vi "Run 03.vi"(11 "NXT/EV3 in":T1) -> (3 "EV3 out":T1)   [LabVIEW 2016]
uses:
  <vilib>/NXT/Subs/LVHSConnector.ctl
  <vilib>/NXT/LegoClasses/BrickReference/BrickReference.lvclass
  <vilib>/NXT/Block Support/NXT_ButtonSelector.ctl
  <vilib>/NXT/Dual Mode Library/Waits/Wait_Btn_Press.vi
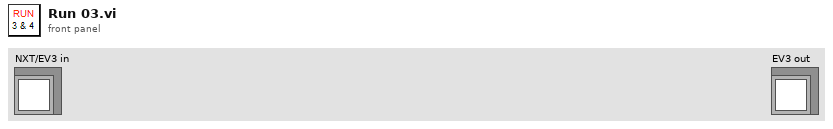
[diagram p1: front panel]
types:
  T1 = typedef "LVHSConnector.ctl" = refnum<class "BrickReference.lvclass">
  T2 = typedef "NXT_ButtonSelector.ctl" = u16
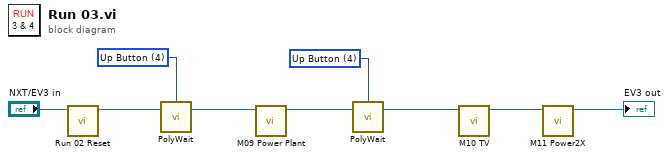
[diagram p0: block diagram]
diagram:
  w5 = T2 4 items=["Enter button"=3, "Left button"=2, "Right button"=1, "Up Button"=4, "Down Button"=5] ("Button (Enter button)")
  w8 = T2 4 items=["Enter button"=3, "Left button"=2, "Right button"=1, "Up Button"=4, "Down Button"=5] ("Button (Enter button)")
  n1 = call "Run 02 Reset.vi"("NXT/EV3 in"="NXT/EV3 in") -> ("NXT/EV3 out"=w7:T1)  [unwired: 10 in]
  n2 = call-poly <vilib>:"PolyWait.vi"("NXT/EV3"=w7, "Button (Enter button)"=w8) -> ("NXT/EV3"=w9:T1)  [unwired: 2 in]
  n3 = call "M09 Power Plant.vi"("EV3 in"=w9) -> ("EV3 out"=w4:T1)  [unwired: 10 in]
  n4 = call-poly <vilib>:"PolyWait.vi"("NXT/EV3"=w4, "Button (Enter button)"=w5) -> ("NXT/EV3"=w3:T1)  [unwired: 2 in]
  n5 = call "M10 TV.vi"("NXT/EV3"=w3) -> ("EV3 out"=w2:T1)  [unwired: 10 in]
  n6 = call "M11 Power2X.vi"("NXT/EV3"=w2) -> ("EV3 out"=→"EV3 out":T1)  [unwired: 10 in]
